vi "InjectionCounter2Steps.vi"(9 "Timestep":dbl=0.1, 10 "Time":dbl=8.0, 11 "NumPoints":dbl=5.0) -> (3 "Array":dbl[](array[numeric]))   [LabVIEW 2016]
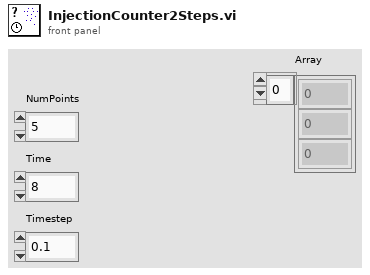
[diagram p1: front panel]
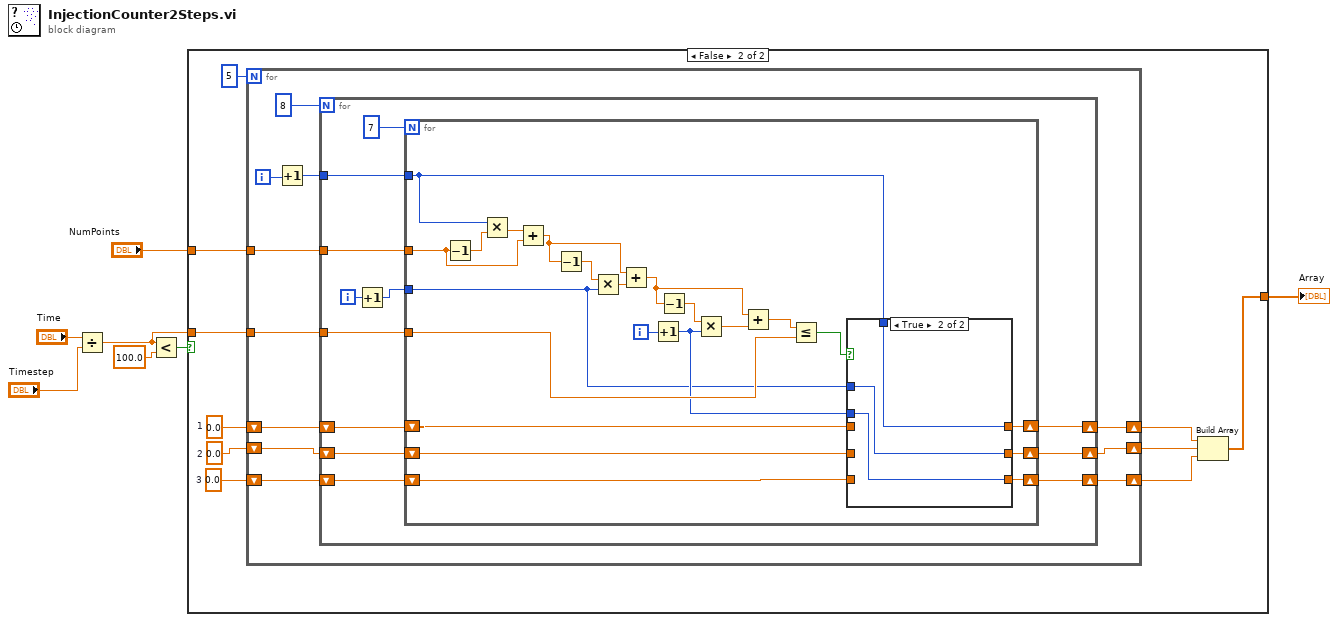
[diagram p0: block diagram]
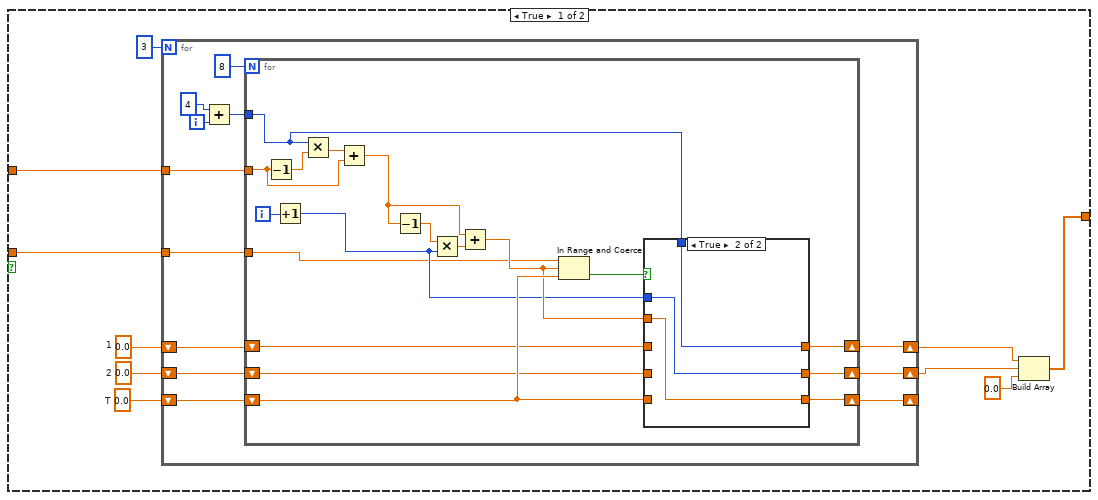
[diagram p2: hidden frame]
diagram:
  n1 = Divide(x="Time", y="Timestep") -> (x/y=w1:dbl)
  n2 = Less?(x=w1, y=100.0) -> (x < y?=w4:bool)
  n3 = case shown="False" w4 {
    tunnel: [w15 w63] -> w3
    tunnel: "NumPoints" -> [w14 w62]
    tunnel: w1 -> [w13 w61]
    frame True {
      w10 = 0.0  # T
      w11 = 0.0  # 2
      w12 = 0.0  # 1
      n4 = for {
        N: 3 -> [_]
        tunnel: w14 -> [w25]
        tunnel: w13 -> [w24]
        shift-right: [w22] -> w9
        shift-left: w12 -> [w23]
        shift-right: [w21] -> w8
        shift-left: w11 -> [w20]
        shift-right: [w19] -> _
        shift-left: w10 -> [w18]
        i -> [w28]
        n5 = Add(x=4, y=w28) -> (x+y=w26:i32)
        n6 = for {
          N: 8 -> [_]
          tunnel: w25 -> [w31]
          tunnel: w24 -> [w30]
          tunnel: w26 -> [w32]
          shift-right: [w36] -> w22
          shift-left: w23 -> [w35]
          shift-right: [w37] -> w21
          shift-left: w20 -> [w38]
          shift-right: [w39] -> w19
          shift-left: w18 -> [w40]
          i -> [w47]
          n7 = Decrement(x=w31) -> (x-1=w46:dbl)
          n8 = Increment(x=w47) -> (x+1=w33:i32)
          n9 = Multiply(x=w32, y=w46) -> (x*y=w45:dbl)
          n10 = Add(x=w45, y=w31) -> (x+y=w42:dbl)
          n11 = Decrement(x=w42) -> (x-1=w44:dbl)
          n12 = Multiply(x=w44, y=w33) -> (x*y=w43:dbl)
          n13 = Add(x=w42, y=w43) -> (x+y=w34:dbl)
          n14 = In Range and Coerce(upper limit=w30, x=w34, lower limit=w40) -> (In Range?=w41:bool)  [unwired: 1 out]
          n15 = case shown="True" w41 {
            tunnel: [w50 w53] -> w39
            tunnel: w40 -> [w50 _]
            tunnel: w38 -> [w49 _]
            tunnel: [w49 w52] -> w37
            tunnel: [w48 w51] -> w36
            tunnel: w35 -> [w48 _]
            tunnel: w34 -> [_ w53]
            tunnel: w33 -> [_ w52]
            tunnel: w32 -> [_ w51]
            frame False {
            }
            frame True {
            }
          }
        }
      }
      n16 = Build Array(w9, w8, 0.0 ("element")) -> (w15:dbl[])
    }
    frame False {
      w58 = 0.0  # 3
      w59 = 0.0  # 2
      w60 = 0.0  # 1
      n17 = for {
        N: 5 -> [_]
        tunnel: w62 -> [w73]
        tunnel: w61 -> [w72]
        shift-right: [w68] -> w57
        shift-left: w60 -> [w71]
        shift-right: [w67] -> w56
        shift-left: w59 -> [w70]
        shift-right: [w64] -> w54
        shift-left: w58 -> [w69]
        i -> [w66]
        n18 = Increment(x=w66) -> (x+1=w65:i32)
        n19 = for {
          N: 8 -> [_]
          tunnel: w73 -> [w85]
          tunnel: w72 -> [w84]
          shift-right: [w82] -> w68
          shift-left: w71 -> [w83]
          shift-right: [w81] -> w67
          shift-left: w70 -> [w80]
          shift-right: [w79] -> w64
          shift-left: w69 -> [w78]
          tunnel: w65 -> [w75]
          i -> [w77]
          n20 = Increment(x=w77) -> (x+1=w76:i32)
          n21 = for {
            N: 7 -> [_]
            tunnel: w85 -> [w96]
            tunnel: w84 -> [w91]
            tunnel: w76 -> [w88]
            shift-right: [w98] -> w82
            shift-left: w83 -> [w97]
            shift-right: [w99] -> w81
            shift-left: w80 -> [w100]
            shift-right: [w101] -> w79
            shift-left: w78 -> [w102]
            tunnel: w75 -> [w87]
            i -> [w108]
            n22 = Decrement(x=w96) -> (x-1=w107:dbl)
            n23 = Multiply(x=w87, y=w107) -> (x*y=w106:dbl)
            n24 = Add(x=w106, y=w96) -> (x+y=w103:dbl)
            n25 = Decrement(x=w103) -> (x-1=w105:dbl)
            n26 = Multiply(x=w105, y=w88) -> (x*y=w104:dbl)
            n27 = Add(x=w103, y=w104) -> (x+y=w93:dbl)
            n28 = Increment(x=w108) -> (x+1=w89:i32)
            n29 = Decrement(x=w93) -> (x-1=w94:dbl)
            n30 = Multiply(x=w94, y=w89) -> (x*y=w95:dbl)
            n31 = Add(x=w93, y=w95) -> (x+y=w92:dbl)
            n32 = Less Or Equal?(x=w92, y=w91) -> (x <= y?=w90:bool)
            n33 = case shown="True" w90 {
              tunnel: [w111 w114] -> w101
              tunnel: w102 -> [w111 _]
              tunnel: w100 -> [w110 _]
              tunnel: [w110 w113] -> w99
              tunnel: [w109 w112] -> w98
              tunnel: w97 -> [w109 _]
              tunnel: w89 -> [_ w114]
              tunnel: w88 -> [_ w113]
              tunnel: w87 -> [_ w112]
              frame False {
              }
              frame True {
              }
            }
          }
        }
      }
      n34 = Build Array(w57, w56, w54) -> (w63:dbl[])
    }
  }
  "Array" <- w3
